vi "PostBuild Action.vi"(8 "error in (no error)":errorcluster, 11 "MGI_TrayIcon in":refnum<class "MGI_TrayIcon.lvclass">) -> (0 "error out":errorcluster, 3 "MGI_TrayIcon out":refnum<class "MGI_TrayIcon.lvclass">)   [LabVIEW 2016, in "MGI_TrayIcon.lvclass"]
doc: "Authored by Derek E. Trepanier\nsupport@mooregoodideas.com\nwww.mooregoodideas.com\n\nCopyright (c) 2012, Moore Good Ideas, Inc.\n\nAll rights reserved.\n\nRedistribution and use in source and binary forms, with or without modification, are permitted provided that the following conditions are met:\n\n * Redistributions of source code must retain the above copyright notice, this list of conditions and the following disclaimer.\n * Redistributions in binary form must reproduce the above copyright notice, this list of conditions and the following disclaimer in the documentation and/or other materials provided with the distribution.\n * Neither the name of Moore Good Ideas, Inc. nor the names of its contributors may be used to endorse or promote products derived from this software without specific prior written permission.\n\nTHIS SOFTWARE IS PROVIDED BY THE COPYRIGHT HOLDERS AND CONTRIBUTORS \"AS IS\" AND ANY EXPRESS OR IMPLIED WARRANTIES, INCLUDING, BUT NOT LIMITED TO, THE IMPLIED WARRANTIES OF MERCHANTABILITY AND FITNESS FOR A PARTICULAR PURPOSE ARE DISCLAIMED. IN NO EVENT SHALL THE COPYRIGHT OWNER OR CONTRIBUTORS BE LIABLE FOR ANY DIRECT, INDIRECT, INCIDENTAL, SPECIAL, EXEMPLARY, OR CONSEQUENTIAL DAMAGES (INCLUDING, BUT NOT LIMITED TO, PROCUREMENT OF SUBSTITUTE GOODS OR SERVICES; LOSS OF USE, DATA, OR PROFITS; OR BUSINESS INTERRUPTION) HOWEVER CAUSED AND ON ANY THEORY OF LIABILITY, WHETHER IN CONTRACT, STRICT LIABILITY, OR TORT (INCLUDING NEGLIGENCE OR OTHERWISE) ARISING IN ANY WAY OUT OF THE USE OF THIS SOFTWARE, EVEN IF ADVISED OF THE POSSIBILITY OF SUCH DAMAGE."
uses:
  <userlib>/_MGI/Menu Building/MenuTypes/TrayIcon/MGI_TrayIcon.lvclass
  <userlib>/_MGI/Menu Building/MenuTypes/TrayIcon/MGI_TrayIcon.lvclass/MGI_TrayIcon.ctl
  System.Drawing
  System.Windows.Forms
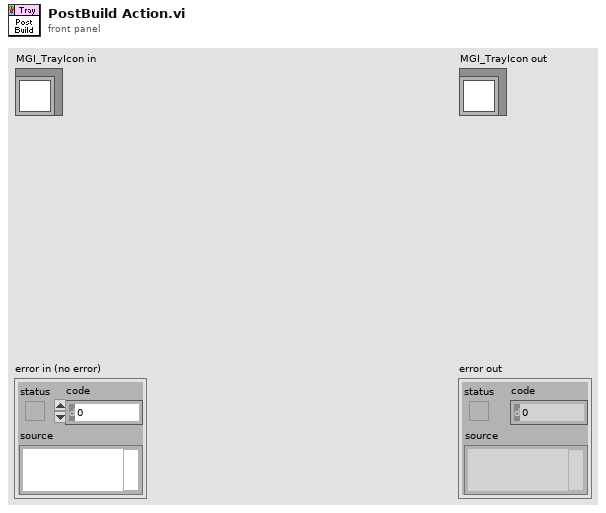
[diagram p1: front panel]
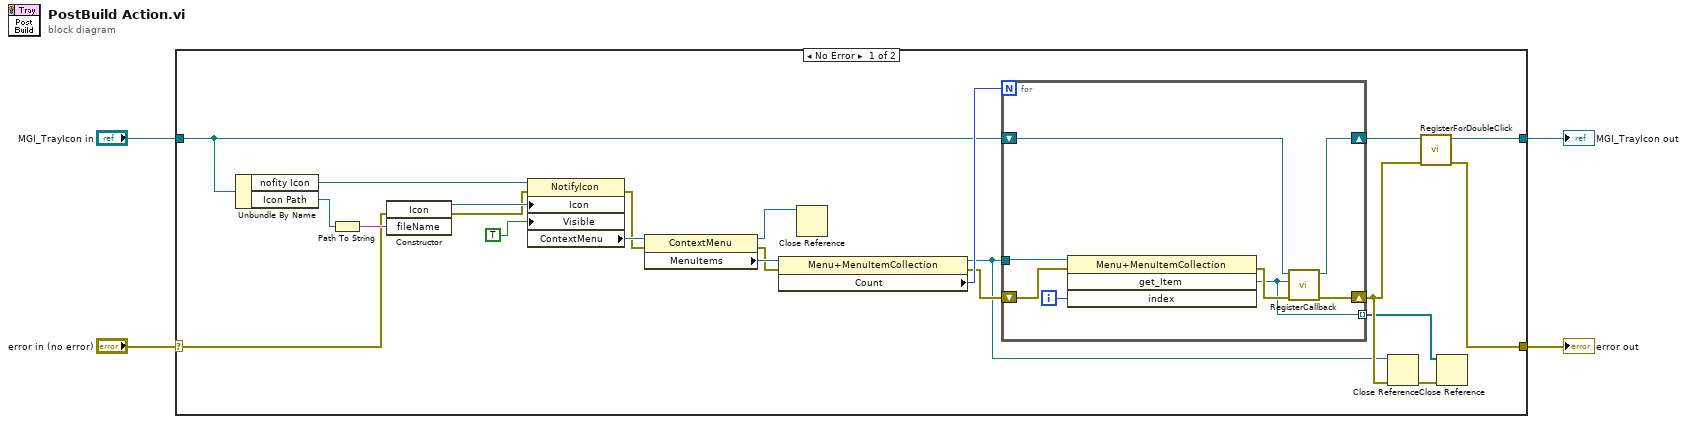
[diagram p0: block diagram]
diagram:
  n1 = case shown="No Error" "error in (no error)" {
    selector: "error in (no error)" -> [w10 w35]
    tunnel: "MGI_TrayIcon in" -> [w20 w36]
    tunnel: [w12 w36] -> w3
    tunnel: [w11 w35] -> w2
    frame No Error {
      n2 = Unbundle By Name(w20) -> ("nofity Icon"=w26:refnum<k24>, "Icon Path"=w15:path)
      n3 = Path To String(path=w15) -> (string=w16:string)
      n4 = constructor class="Icon"(error in=w10, "fileName"=w16) -> (reference out=w24:refnum<k24>, error out=w14:errorcluster)  [unwired: 2 in, 2 out]
      n5 = property class="NotifyIcon"(reference=w26, error in=w14, "Icon"=w24, "Visible"=TRUE) -> (error out=w17:errorcluster, "ContextMenu"=w23:refnum<k24>)  [unwired: 1 out]
      n6 = property class="ContextMenu"(reference=w23, error in=w17) -> (reference out=w9:refnum<k24>, error out=w18:errorcluster, "MenuItems"=w21:refnum<k24>)
      n7 = property class="Menu+MenuItemCollection"(reference=w21, error in=w18) -> (reference out=w7:refnum<k24>, error out=w19:errorcluster, "Count"=w22:i32)
      n8 = Close Reference(reference=w9) -> ()  [unwired: 1 in, 1 out]
      n9 = for {
        N: w22 -> [_]
        tunnel: w7 -> [w34]
        shift-right: [w31] -> w13
        shift-left: w20 -> [w32]
        shift-right: [w30] -> w8
        shift-left: w19 -> [w29]
        tunnel: [w27] -> w5 mode=indexing
        i -> [w33]
        n10 = invoke class="Menu+MenuItemCollection" method="get_Item"(reference=w34, error in=w29, "index"=w33) -> (error out=w28:errorcluster, "get_Item"=w27:refnum<k24>)  [unwired: 1 in, 2 out]
        n11 = call <userlib>:"RegisterCallback.vi"("error in (no error)"=w28, "Menu Item"=w27, "MGI_TrayIcon in"=w32) -> ("error out"=w30:errorcluster, "MGI_TrayIcon out"=w31:refnum<class "MGI_TrayIcon.lvclass">)  [unwired: 7 in]
      }
      n12 = Close Reference(reference=w7, error in (no error)=w8) -> (error out=w6:errorcluster)
      n13 = call <userlib>:"RegisterForDoubleClick.vi"("error in (no error)"=w8, "MGI_TrayIcon in"=w13) -> ("error out"=w11:errorcluster, "MGI_TrayIcon out"=w12:refnum<class "MGI_TrayIcon.lvclass">)  [unwired: 8 in]
      n14 = Close Reference(reference=w5, error in (no error)=w6) -> ()  [unwired: 1 out]
    }
    frame Error {
    }
  }
  "error out" <- w2
  "MGI_TrayIcon out" <- w3
